vi "SVT Crest Factor.vi"   [LabVIEW 2017]
doc: "Computes the crest factor, peak level, and RMS level of <B>scaled signal [EU]</B>. You can use this polymorphic VI to compute the crest factor for a single channel or for N channels. The data type you wire to the <B>scaled signal [EU]</B> input determines the polymorphic instance to use."
uses:
  <vilib>/addons/Sound and Vibration/svt_Level/SoundVib_VibrationLevel.lvlib
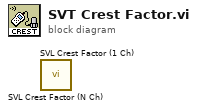
[diagram p0: block diagram]
diagram:
  n1 = call <vilib>:"SVL Crest Factor (N Ch).vi"() -> ()  [unwired: 8 in, 4 out]
  n2 = call <vilib>:"SVL Crest Factor (1 Ch).vi"() -> ()  [unwired: 8 in, 4 out]
